vi "startcase.vi"() -> ()   [LabVIEW 2015]
panel:
  out "lowercase":string
  out "uppercase":string
  out "start case":string
  out "concatenated string 2":string
  out "concatenated string":string
  out "substring 2":string
  out "substring":string
  out "substring before match":string
  in  "String":string
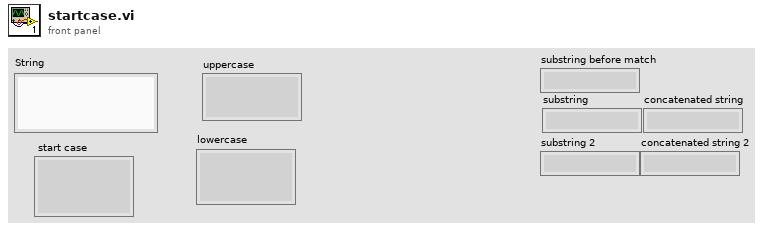
[diagram p1: front panel]
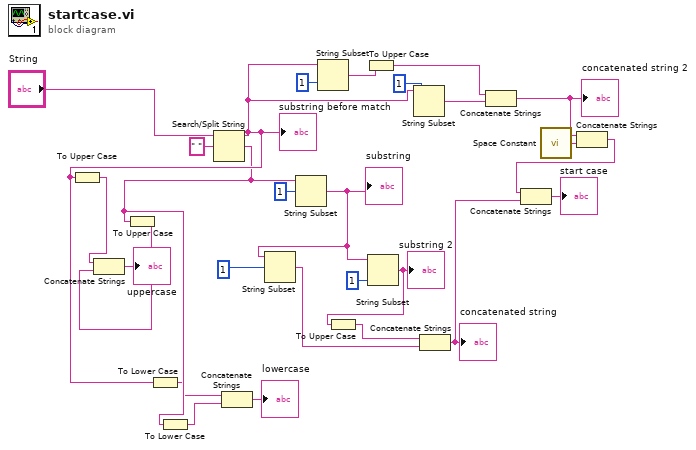
[diagram p0: block diagram]
diagram:
  n1 = Search/Split String(string="String", search string/char (-)=" ") -> (substring before match=w5:string, match + rest of string=w4:string)  [unwired: 1 in, 1 out]
  "substring before match" <- w5
  n2 = To Upper Case(1:w5) -> (0:w8:string)
  n3 = To Upper Case(1:w4) -> (0:w7:string)
  n4 = Concatenate Strings(w8, w7) -> (→"uppercase":string)
  n5 = To Lower Case(string=w5) -> (all lower case string=w3:string)
  n6 = To Lower Case(string=w4) -> (all lower case string=w2:string)
  n7 = Concatenate Strings(w3, w2) -> (→"lowercase":string)
  n8 = String Subset(string=w4, offset (0)=1) -> (substring=w20:string)  [unwired: 1 in]
  "substring" <- w20
  n9 = String Subset(string=w20, offset (0)=1) -> (substring=w21:string)  [unwired: 1 in]
  n10 = String Subset(string=w5, length (rest)=1 ("length (rest)")) -> (substring=w18:string)  [unwired: 1 in]
  n11 = To Upper Case(1:w18) -> (0:w16:string)
  n12 = String Subset(string=w20, length (rest)=1 ("length (rest)")) -> (substring=w24:string)  [unwired: 1 in]
  "substring 2" <- w24
  n13 = To Upper Case(1:w24) -> (0:w22:string)
  n14 = String Subset(string=w5, offset (0)=1) -> (substring=w15:string)  [unwired: 1 in]
  n15 = Concatenate Strings(w22, w21) -> (w14:string)
  "concatenated string" <- w14
  n16 = Concatenate Strings(w16, w15) -> (w11:string)
  "concatenated string 2" <- w11
  n17 = call <vilib>:"Space Constant.vi"() -> ("String"=w10:string)
  n18 = Concatenate Strings(w11, w10) -> (w12:string)
  n19 = Concatenate Strings(w12, w14) -> (→"start case":string)
